vi "Write To Spreadsheet File Mod.vi"(0 "delimiter (Tab)":string="\t", 1 "transpose? (no:F)":bool, 4 "format (%.3f)":string="%.3f", 5 "append to file? (new file:F)":bool, 6 "1D data":dbl[](array[numeric]) format="%.2f", 7 "2D data":dbl[][](array[numeric]) format="%.2f", 8 "file path (dialog if empty)":path) -> (3 "new file path (Not A Path if cancelled)":path)   [LabVIEW 2014]
doc: "Converts a 2D or 1D array of single-precision (SGL) numbers to a text string and writes the string to a new byte stream file or appends the string to an existing file.\n\nChanged to take DBL instead of SGL. / RoSt"
panel:
  in  "prompt":string="Choose file to write."
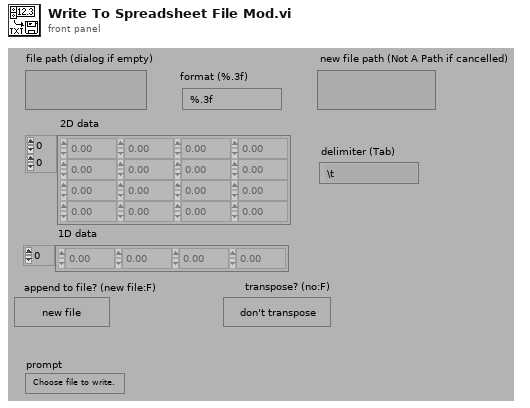
[diagram p1: front panel]
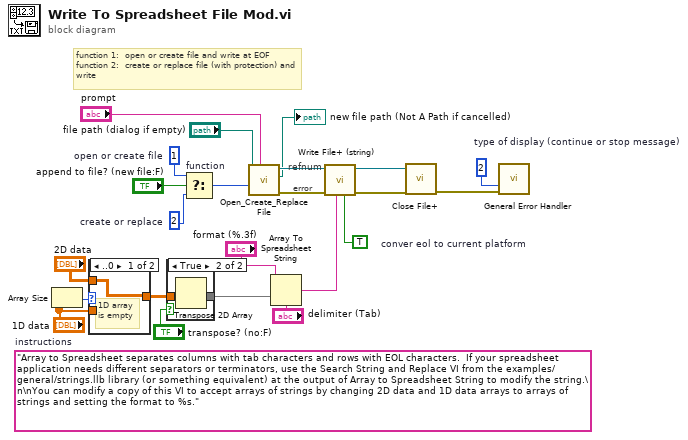
[diagram p0: block diagram]
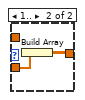
[diagram p3: hidden frame]
diagram:
  (unwired) "Array to Spreadsheet separates columns with tab characters and rows with EOL characters.  If your spreadsheet application needs different separators or terminators, use the Search String and Replace VI from the examples/general/strings.llb library (or something equivalent) at the output of Array to Spreadsheet String to modify the string.\n\nYou can modify a copy of this VI to accept arrays of strings by changing 2D data and 1D data arrays to arrays of strings and setting the format to %s."  # instructions
  w3 = i16 2  # create or replace
  w6 = TRUE  # conver eol to current platform
  w21 = 2  # type of display (continue or stop message)
  w22 = i16 1  # open or create file
  # "error"
  # "refnum"
  # "function 1:  open or create file and write at EOF\nfunction 2:  create or replace file (with protection) and write"
  n1 = Array Size(array="1D data") -> (size(s)=w19:i32)
  n2 = case shown="..0" w19 {
    tunnel: "1D data" -> [_ w26]
    tunnel: [w24 w25] -> w15
    tunnel: "2D data" -> [w24 _]
    frame ..0 {
      # "1D array is empty"
    }
    frame 1.. {
      n3 = Build Array(w26) -> (w25:dbl[][])
    }
  }
  n4 = case shown="True" "transpose? (no:F)" {
    tunnel: [w27 w29] -> w13
    tunnel: w15 -> [w27 w28]
    frame False {
    }
    frame True {
      n5 = Transpose 2D Array(2D array=w28) -> (transposed array=w29:dbl[][])
    }
  }
  n6 = Select "function"(t=w22, s="append to file? (new file:F)", f=w3) -> (s? t:f=w12:i16)
  n7 = call <vilib>:"Open_Create_Replace File.vi"("prompt"="prompt", "function (open:0)"=w12, "file path"="file path (dialog if empty)") -> ("error out"=w10:errorcluster, "new file path"=→"new file path (Not A Path if cancelled)":path, "refnum"=w5:refnum<file>)  [unwired: 5 in, 1 out]
  n8 = Array To Spreadsheet String(delimiter (Tab)="delimiter (Tab)", array=w13, 3:"format (%.3f)") -> (spreadsheet string=w9:string)
  n9 = call <vilib>:"Write File+ (string).vi"("convert eol? (no:F)"=w6, "string"=w9, "error in (no error)"=w10, "refnum"=w5) -> ("error out"=w20:errorcluster, "dup refnum"=w8:refnum<file>)  [unwired: 3 in, 1 out]
  n10 = call <vilib>:"Close File+.vi"("error in (no error)"=w20, "refnum"=w8) -> ("error out"=w7:errorcluster)  [unwired: 3 in, 2 out]
  n11 = call <vilib>:"General Error Handler.vi"("type of dialog (OK msg:1)"=w21, "error in (no error)"=w7) -> ()  [unwired: 9 in, 5 out]
